vi "RgbaToU32_1D.vi"(11 "Rgba":T1[](array[typedef])) -> (3 "U32":u32[](array[numeric]))   [LabVIEW 2020, in "OpenLvVision_Image.lvlib" / "DataAccess.lvlib"]
doc: "Convert an color cluster into an number"
uses:
  DataAccess.lvlib
  TypeDef/RgbaU32.ctl
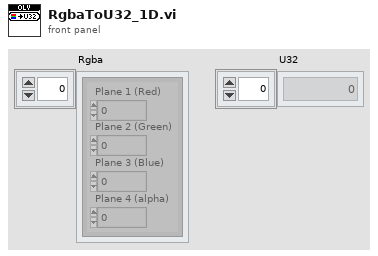
[diagram p1: front panel]
types:
  T1 = typedef "OpenLvVision_Image.lvlib/DataAccess.lvlib/RgbaU32.ctl" = cluster{"Plane 1 (Red)":u8, "Plane 2 (Green)":u8, "Plane 3 (Blue)":u8, "Plane 4 (alpha)":u8}
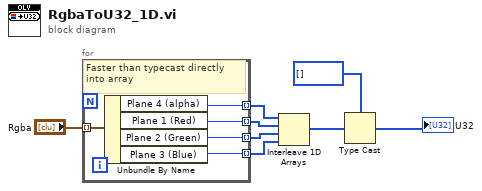
[diagram p0: block diagram]
diagram:
  n1 = for {
    tunnel: "Rgba" -> [w13] mode=indexing
    tunnel: [w12] -> w7 mode=indexing
    tunnel: [w11] -> w5 mode=indexing
    tunnel: [w10] -> w6 mode=indexing
    tunnel: [w9] -> w4 mode=indexing
    # "Faster than typecast directly into array"
    n2 = Unbundle By Name(w13) -> ("Plane 4 (alpha)"=w12:u8, "Plane 1 (Red)"=w11:u8, "Plane 2 (Green)"=w10:u8, "Plane 3 (Blue)"=w9:u8)
  }
  n3 = Interleave 1D Arrays(w7, w5, w6, w4) -> (w3:u8[])
  n4 = Type Cast(type=u32[] [], x=w3) -> (*(type *) &x=→"U32":u32[])
